vi "Create Cell Range.vi"(8 "error in":errorcluster, 11 "Cell Range":string) -> (0 "error out":errorcluster, 3 "Cell Range":string[][](array[string]))   [LabVIEW 2021, in "Open Xml.lvlib"]
uses:
  Open Xml.lvlib
  <vilib>/Analysis/1siggen.llb/Ramp Pattern by Delta.vi
  <vilib>/Analysis/NI_AALBase.lvlib
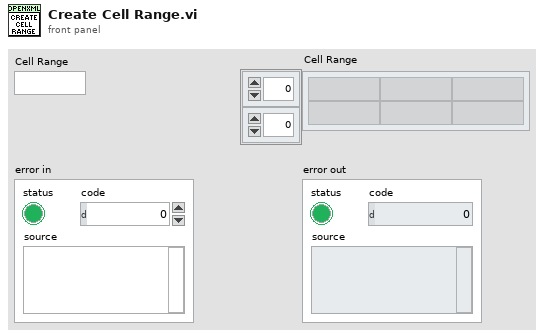
[diagram p1: front panel]
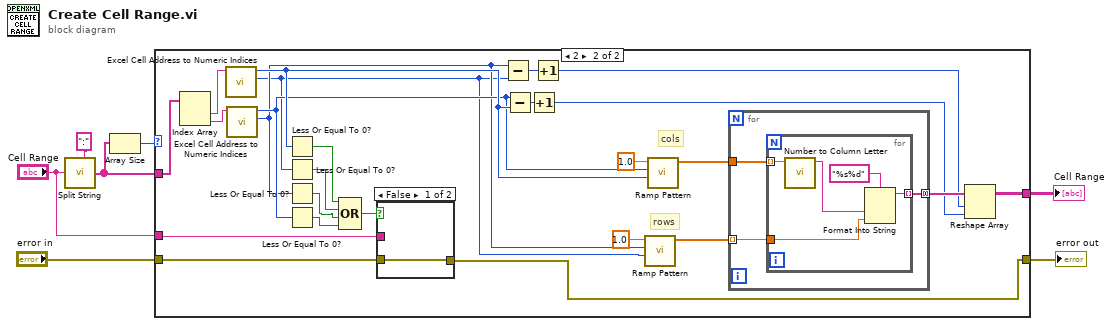
[diagram p0: block diagram]
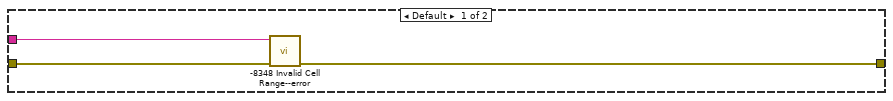
[diagram p2: hidden frame]
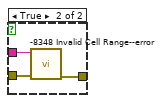
[diagram p3: hidden frame]
diagram:
  n1 = call <vilib>:"Split String.vi"("Split Pattern"=":", "Input String"="Cell Range") -> ("Split String"=w6:string[])  [unwired: 5 in]
  n2 = Array Size(array=w6) -> (size(s)=w5:i32)
  n3 = case shown="2" w5 {
    tunnel: w6 -> [_ w30]
    tunnel: "error in" -> [w10 w21]
    tunnel: [w9 w11] -> w3
    tunnel: "Cell Range" -> [w8 w17]
    tunnel: [_ w27] -> w1
    frame Default {
      n4 = call "-8348 Invalid Cell Range--error.vi"("error in"=w10, "Argument"=w8) -> ("error out"=w9:errorcluster)  [unwired: 9 in]
    }
    frame 2 {
      # "rows"
      # "cols"
      n5 = Index Array(array=w30) -> (element #1=w29:string, element #2=w28:string)  [unwired: 2 in]
      n6 = call "Excel Cell Address to Numeric Indices.vi"("Cell Name"=w29) -> ("Row Number"=w12:i32, "Column Number"=w15:i32)  [unwired: 9 in]
      n7 = call "Excel Cell Address to Numeric Indices.vi"("Cell Name"=w28) -> ("Row Number"=w13:i32, "Column Number"=w14:i32)  [unwired: 9 in]
      n8 = Less Or Equal To 0?(x=w15) -> (x <= 0?=w18:bool)
      n9 = Less Or Equal To 0?(x=w12) -> (x <= 0?=w19:bool)
      n10 = Less Or Equal To 0?(x=w13) -> (x <= 0?=w20:bool)
      n11 = Less Or Equal To 0?(x=w14) -> (x <= 0?=w22:bool)
      n12 = Compound Arithmetic op=OR(w18, w19, w20, w22) -> (w16:bool)
      n13 = case shown="False" w16 {
        tunnel: w21 -> [w36 w39]
        tunnel: w17 -> [_ w38]
        tunnel: [w36 w37] -> w11
        frame False {
        }
        frame True {
          n14 = call "-8348 Invalid Cell Range--error.vi"("error in"=w39, "Argument"=w38) -> ("error out"=w37:errorcluster)  [unwired: 9 in]
        }
      }
      n15 = Subtract(x=w13, y=w12) -> (x-y=w26:i32)
      n16 = Subtract(x=w14, y=w15) -> (x-y=w25:i32)
      n17 = Increment(x=w25) -> (x+1=w23:i32)
      n18 = Increment(x=w26) -> (x+1=w24:i32)
      n19 = call-poly <vilib>:"Ramp Pattern.vi"("start"=w12, "end"=w13, "delta"=1.0) -> ("Ramp Pattern"=w31:dbl[])  [unwired: 6 in, 2 out]
      n20 = call-poly <vilib>:"Ramp Pattern.vi"("start"=w15, "end"=w14, "delta"=1.0) -> ("Ramp Pattern"=w32:dbl[])  [unwired: 6 in, 2 out]
      n21 = for {
        tunnel: [w41] -> w35 mode=concatenating
        tunnel: w32 -> [w40]
        tunnel: w31 -> [w42] mode=indexing
        n22 = for {
          tunnel: w42 -> [w46]
          tunnel: [w45] -> w41 mode=indexing
          tunnel: w40 -> [w44] mode=indexing
          n23 = call "Number to Column Letter.vi"("Number"=w44) -> ("Letter"=w43:string)  [unwired: 10 in]
          n24 = Format Into String(format string="%s%d", w43, w46) -> (resulting string=w45:string)  [unwired: 2 in, 1 out]
        }
      }
      n25 = Reshape Array(w35, w24, w23) -> (w27:string[][])
    }
  }
  "error out" <- w3
  "Cell Range" <- w1
